vi "Configure Trigger (Pulse).vi"(0 "VISA resource name":refnum<visa-resource-name>, 2 "Upper Limit (2E-6 s)":dbl=2e-06, 5 "Source (1: Channel 1)":i32(ring)=1 items=["Channel 1"=1, "Channel 2"=2, "Channel 3"=3, "Channel 4"=4], 7 "Trigger Condition (0: Positive Greater)":i32(ring) items=["Positive Greater", "Positive Less", "Negative Greater", "Negative Less", "Positive Greater Less", "Negative Greater Less"], 11 "error in (no error)":errorcluster, 13 "Lower Limit (1E-6 s)":dbl=1e-06, 14 "Level (0)":dbl) -> (4 "VISA resource name out":refnum<visa-resource-name>, 15 "error out":errorcluster)   [LabVIEW 2015, in "ZhiYuan ZDS Series for TCP.lvlib"]
doc: "Configures the setting for pulse trigger."
uses:
  ZhiYuan ZDS Series for TCP.lvlib
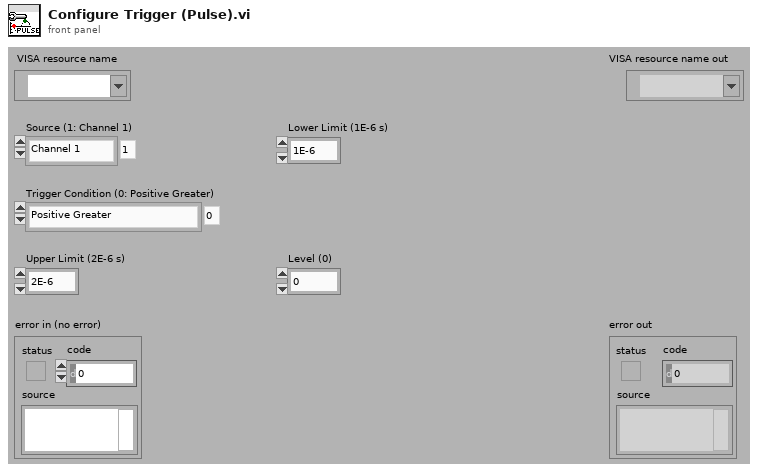
[diagram p1: front panel]
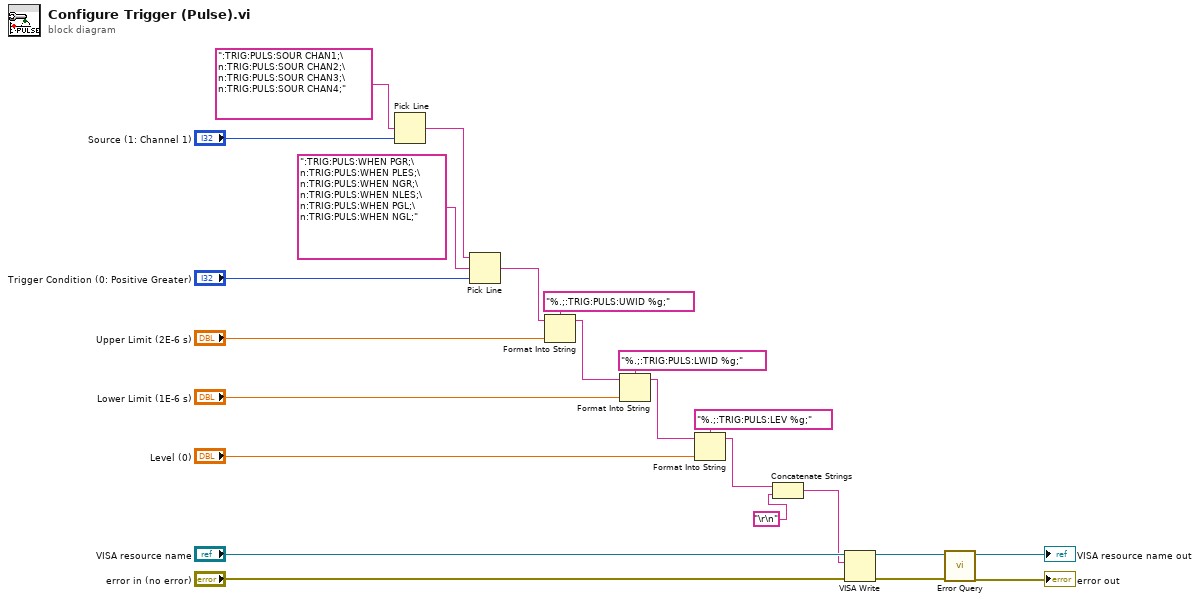
[diagram p0: block diagram]
diagram:
  n1 = Pick Line(multi-line string=":TRIG:PULS:SOUR CHAN1;\n:TRIG:PULS:SOUR CHAN2;\n:TRIG:PULS:SOUR CHAN3;\n:TRIG:PULS:SOUR CHAN4;", line index="Source (1: Channel 1)") -> (output string=w19:string)  [unwired: 1 in]
  n2 = Pick Line(string ("")=w19, multi-line string=":TRIG:PULS:WHEN PGR;\n:TRIG:PULS:WHEN PLES;\n:TRIG:PULS:WHEN NGR;\n:TRIG:PULS:WHEN NLES;\n:TRIG:PULS:WHEN PGL;\n:TRIG:PULS:WHEN NGL;", line index="Trigger Condition (0: Positive Greater)") -> (output string=w18:string)
  n3 = Format Into String(format string="%.;:TRIG:PULS:UWID %g;", initial string=w18, "Upper Limit (2E-6 s)") -> (resulting string=w15:string)  [unwired: 1 in, 1 out]
  n4 = Format Into String(format string="%.;:TRIG:PULS:LWID %g;", initial string=w15, "Lower Limit (1E-6 s)") -> (resulting string=w12:string)  [unwired: 1 in, 1 out]
  n5 = Format Into String(format string="%.;:TRIG:PULS:LEV %g;", initial string=w12, "Level (0)") -> (resulting string=w3:string)  [unwired: 1 in, 1 out]
  n6 = Concatenate Strings(w3, "\r\n") -> (w2:string)
  n7 = VISA Write(VISA resource name="VISA resource name", write buffer=w2, error in (no error)="error in (no error)") -> (VISA resource name out=w7:refnum<visa-resource-name>, error out=w6:errorcluster)  [unwired: 1 out]
  n8 = call "Error Query.vi"("error in (no error)"=w6, "VISA resource name"=w7) -> ("error out"=→"error out":errorcluster, "VISA resource name out"=→"VISA resource name out":refnum<visa-resource-name>)  [unwired: 6 in, 2 out]
